vi "Write NChan NSamp 2D SGL.vi"(8 "error in (no error)":errorcluster, 10 "data":sgl[][](array[numeric]), 11 "Analog Output in":refnum<class "Analog output.lvclass">) -> (0 "error out":errorcluster, 3 "Analog Output out":refnum<class "Analog output.lvclass">)   [LabVIEW 2009, in "MicroDAQ.lvlib" / "Analog output.lvclass"]
doc: "Writes buffor of floating-points samples to all channels."
uses:
  <instrlib>/MicroDAQ/Channel/Analog Output/Analog output.lvclass
  <instrlib>/MicroDAQ/Channel/Analog Output/Analog output.lvclass/Analog output.ctl
  <instrlib>/MicroDAQ/Channel/Channel.lvclass
  <instrlib>/MicroDAQ/Mlink library wraper/mlink.lvlib
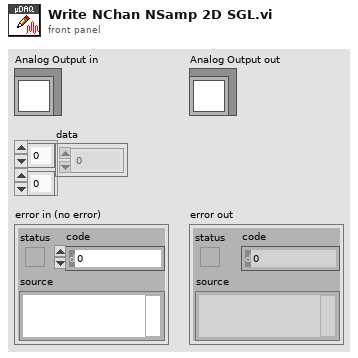
[diagram p1: front panel]
types:
  T1 = enum16{"non-blocking / no index reset", "blocking / index reset"}
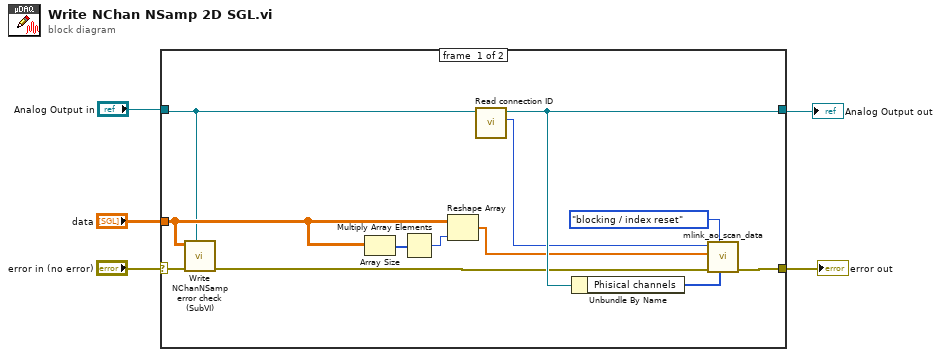
[diagram p0: block diagram]
diagram:
  n1 = case shown="No Error" "error in (no error)" {
    selector: "error in (no error)" -> [w9 w19]
    tunnel: [w14 w19] -> w4
    tunnel: [w17 w18] -> w1
    tunnel: "Analog Output in" -> [w6 w18]
    tunnel: "data" -> [w7 _]
    frame #0 {
      n2 = call <instrlib>:"Write NChanNSamp error check (SubVI).vi"("Analog output in"=w6, "error in (no error)"=w9, "data"=w7) -> ("error out"=w8:errorcluster)  [unwired: 8 in]
      n3 = Array Size(array=w7) -> (size(s)=w16:i32[])
      n4 = Multiply Array Elements(1:w16) -> (0:w15:i32)
      n5 = Reshape Array(w7, w15) -> (w10:sgl[])
      n6 = call <instrlib>:"Read connection ID.vi"("Task in"=w6) -> ("connection ID"=w13:i32, "Task out"=w17:refnum<class "Analog output.lvclass">)  [unwired: 9 in]
      n7 = Unbundle By Name(w17) -> ("Phisical channels"=w11:u8[])
      n8 = call <instrlib>:"mlink_ao_scan_data.vi"("channels"=w11, "opt"=T1."blocking / index reset", "error in (no error)"=w8, "data"=w10, "connection ID"=w13) -> ("error out"=w14:errorcluster)  [unwired: 5 in, 1 out]
    }
    frame #1 {
    }
  }
  "error out" <- w4
  "Analog Output out" <- w1
